vi "test - Refnum.vi"(8 "error in (no error)":errorcluster, 11 "TestCase in":refnum<class "testcase-Supported-Datatype.lvclass">) -> (0 "error out":errorcluster, 3 "TestCase out":refnum<class "testcase-Supported-Datatype.lvclass">)   [LabVIEW 2017, in "testcase-Supported-Datatype.lvclass"]
uses:
  testcase-Supported-Datatype.lvclass
  4933ebb4-187b-4d02-a477-b811f479a1ff.vi
  38b0d59b-7d4c-4ce6-bed7-fc6aed411a90.vi
  addons/API-String-Arugments-Support/_Support/Data To API String Arguments.vi
  addons/API-String-Arugments-Support/_Support/Convert API String Arguments to Data(variant).vi
  <vilib>/addons/_JKI Toolkits/VI Tester/TestCase.llb/TestCase.lvclass
  C:/Program Files (x86)/National Instruments/LabVIEW 2017/vi.lib/addons/_JKI Toolkits/VI Tester/TestCase.llb/TestCase.lvclass
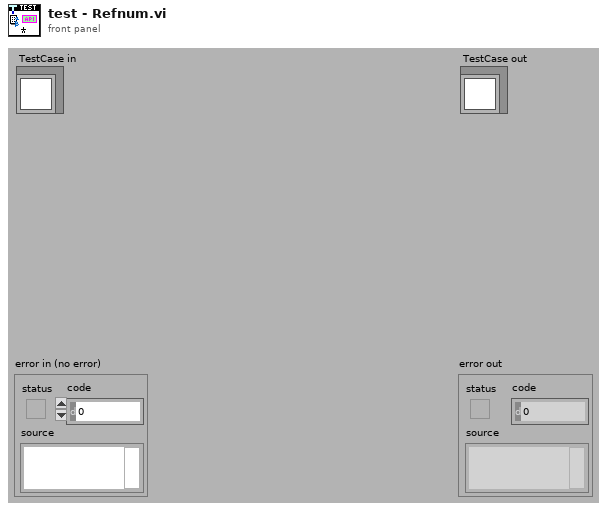
[diagram p1: front panel]
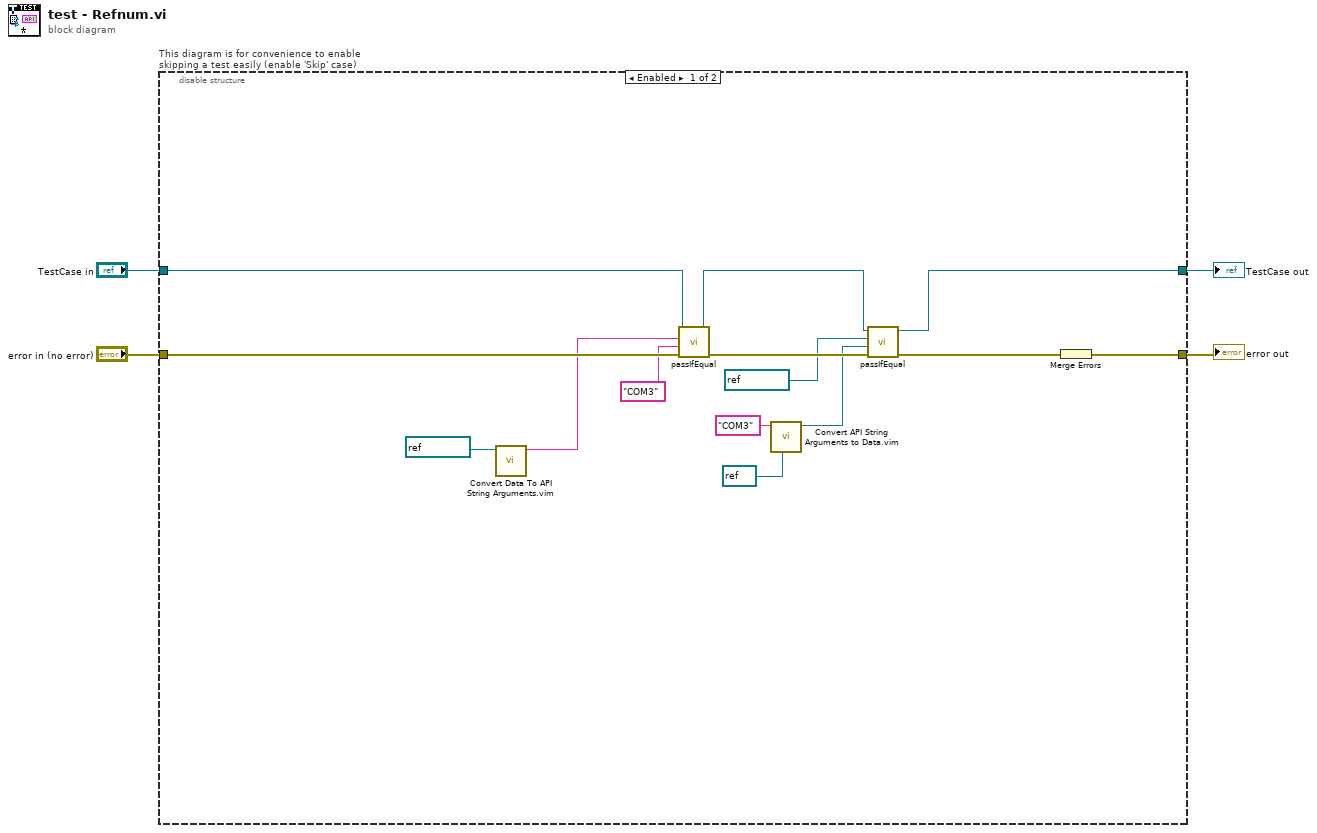
[diagram p0: block diagram]
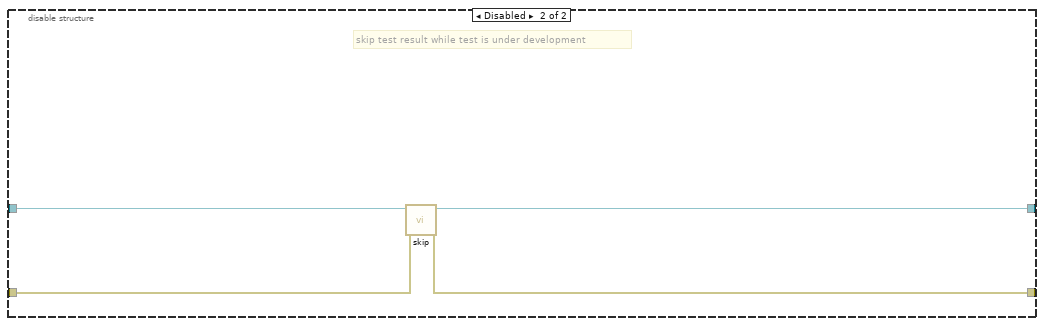
[diagram p2: hidden frame]
diagram:
  n1 = disable-structure "This diagram is for convenience to enable skipping a test easily (enable 'Skip' case)" shown="Enabled" {
    disable-tunnel: "TestCase in" -> [w18 w22]
    disable-tunnel: [w11 w20] -> w1
    disable-tunnel: [w17 w21] -> w3
    disable-tunnel: "error in (no error)" -> [w16 w19]
    frame Enabled {
      n2 = call "Convert Data To API String Arguments.vim"("Data"=refnum<visa-resource-name> "COM3" ("VISA resource name")) -> ("API String"=w14:string)  [unwired: 7 in, 1 out]
      n3 = call-dynamic "passIfEqual.vi"("error in (no error)"=w16, "y"="COM3" ("String"), "x"=w14, "TestCase in"=w18) -> ("error out"=w9:errorcluster, "TestCase out"=w12:refnum<class "testcase-Supported-Datatype.lvclass">)  [unwired: 6 in]
      n4 = call "Convert API String Arguments to Data.vim"("Reference Type"=refnum<visa-resource-name> refnum ("VISA resource name"), "API String"="COM3" ("String")) -> ("Data"=w5:refnum<visa-resource-name>)  [unwired: 6 in, 1 out]
      n5 = call-dynamic "passIfEqual.vi"("error in (no error)"=w9, "y"=w5, "x"=refnum<visa-resource-name> "COM3" ("VISA resource name"), "TestCase in"=w12) -> ("error out"=w10:errorcluster, "TestCase out"=w11:refnum<class "testcase-Supported-Datatype.lvclass">)  [unwired: 6 in]
      n6 = Merge Errors(w10) -> (w17:errorcluster)
    }
    frame Disabled {
      # "skip test result while test is under development"
      n7 = call <vilib>:"skip.vi"("error in (no error)"=w19, "TestCase in"=w22) -> ("error out"=w21:errorcluster, "TestCase out"=w20:refnum<class "testcase-Supported-Datatype.lvclass">)  [unwired: 8 in]
    }
  }
  "error out" <- w3
  "TestCase out" <- w1
